vi "I2C Close.vi"(7 "I2C Channel (0)":u8, 8 "Error In":errorcluster, 11 "LINX Resource":T1) -> (0 "Error Out":errorcluster, 3 "LINX Resource":T1)   [LabVIEW 2020, in "LMH-LINX.lvlib"]
doc: "Close the specified I2C channel. Not all devices support or require this fuction. Most Wiring (Arduino) comaptible devices do not support this function. \n\nIf the current device does not support this function it will return a 'Function Not Supported' warning which should be handled by the users code."
uses:
  LMH-LINX.lvlib
  Private/Type Defs/LINX Ref.ctl
  Private/Type Defs/Platform.ctl
  Private/Type Defs/Interface.ctl
  Private/Device/Type Defs/LINX Device Config.ctl
  Private/Device/Type Defs/TCP Config.ctl
  Private/Device/Type Defs/Channels.ctl
  Private/Type Defs/Peripheral.ctl
  Private/Utilties/Generate Error.vi
  Private/Device/Device.lvlib
  Private/Local IO/Local IO.lvlib
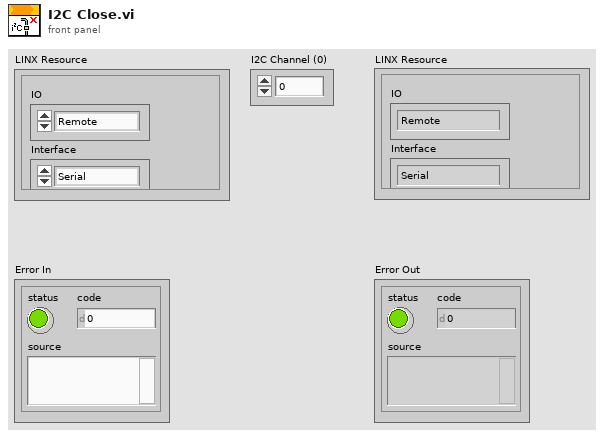
[diagram p1: front panel]
types:
  T1 = typedef "LMH-LINX.lvlib/LINX Ref.ctl" = cluster{"IO":T2, "Interface":T3, "LINX Device Config":T4}
  T2 = typedef "LMH-LINX.lvlib/Platform.ctl" = enum16{"Remote", "Local"}
  T3 = typedef "LMH-LINX.lvlib/Interface.ctl" = enum16{"Serial", "TCP"}
  T4 = typedef "LMH-LINX.lvlib/Device.lvlib/LINX Device Config.ctl" = cluster{"Interface":T3, "COM Port":refnum<visa-resource-name>, "TCP Configuration":T5, "Device Family":u8, "Device ID":u8, "Device Name":string, "TCP Ref":refnum<k5>, "Channels":T6}
  T5 = typedef "LMH-LINX.lvlib/Device.lvlib/TCP Config.ctl" = cluster{"IP Address":string, "Port":u16}
  T6 = typedef "LMH-LINX.lvlib/Channels.ctl" = cluster{"DI":u8[], "DO":u8[], "AI":u8[], "AO":u8[], "PWM":u8[], "QE":u8[], "UART":u8[], "I2C 2":u8[], "SPI":u8[], "CAN":u8[], "Servo":u8[], "AI Ref (V)":dbl, "AI Resolution (Bits)":u8, "AO Ref (V)":dbl, "AO Resolution (Bits)":u8}
  T7 = typedef "LMH-LINX.lvlib/Peripheral.ctl" = enum8{"DI", "DO", "AI", "AO", "PWM", "QE", "UART", "I2C", "SPI", "CAN", "Servo"}
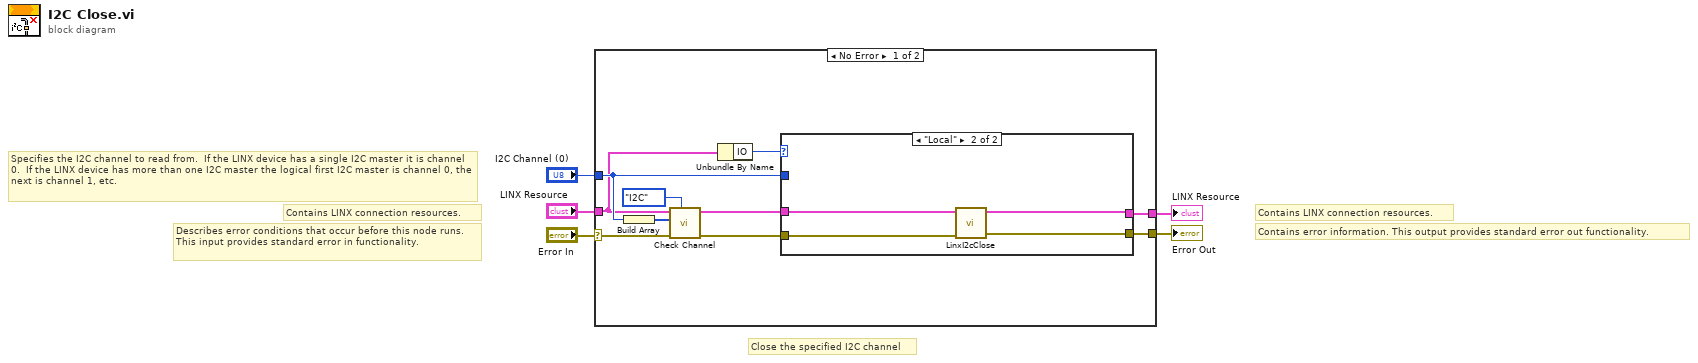
[diagram p0: block diagram]
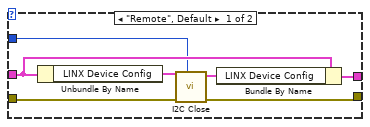
[diagram p2: hidden frame]
diagram:
  # "Specifies the I2C channel to read from.  If the LINX device has a single I2C master it is channel 0.  If the LINX device has more than one I2C master the logical first I2C master is channel 0, the next is channel 1, etc."
  # "Contains LINX connection resources."
  # "Contains error information. This output provides standard error out functionality."
  # "Contains LINX connection resources."
  # "Describes error conditions that occur before this node runs. This input provides standard error in functionality."
  # "Close the specified I2C channel"
  n1 = case shown="No Error" "Error In" {
    selector: "Error In" -> [w6 w28]
    tunnel: [w14 w28] -> w5
    tunnel: [w13 w27] -> w4
    tunnel: "I2C Channel (0)" -> [w9 _]
    tunnel: "LINX Resource" -> [w8 w27]
    frame No Error {
      n2 = Build Array(w9) -> (w12:u8[])
      n3 = call "Check Channel.vi"("Peripheral"=Peripheral."I2C", "Error In"=w6, "Channels"=w12, "LINX Resource"=w8) -> ("Error Out"=w10:errorcluster, "LINX Resource"=w7:T1)  [unwired: 5 in, 1 out]
      n4 = Unbundle By Name(w8) -> ("IO"=w15:T2)
      n5 = case shown="\"Local\"" w15 {
        tunnel: w10 -> [w17 w23]
        tunnel: w7 -> [w22 w26]
        tunnel: [w16 w24] -> w14
        tunnel: [w21 w25] -> w13
        tunnel: w9 -> [w18 _]
        frame "Remote", Default {
          n6 = Unbundle By Name(w22) -> ("LINX Device Config"=w20:T4)
          n7 = call "I2C Close.vi"("I2C Channel"=w18, "Error In"=w17, "LINX Device Config"=w20) -> ("Error Out"=w16:errorcluster, "LINX Device Config"=w19:T4)  [unwired: 7 in]
          n8 = Bundle By Name(cluster=w22, "LINX Device Config"=w19) -> (w21:T1)
        }
        frame "Local" {
          n9 = call "LinxI2cClose.vi"("Error In"=w23, "LINX Resource"=w26) -> ("Error Out"=w24:errorcluster, "LINX Resource"=w25:T1)  [unwired: 8 in]
        }
      }
    }
    frame Error {
    }
  }
  "Error Out" <- w5
  "LINX Resource" <- w4
